vi "begin5RobotsPassGamePlay.vi"(8 "error in (no error)":errorcluster, 10 "Game in":refnum<class "Game.lvclass">, 11 "5RobotsPassGamePlay in":refnum<class "5RobotsPassGamePlay.lvclass">) -> (0 "error out":errorcluster, 1 "Game out":refnum<class "Game.lvclass">, 2 "begin":bool, 3 "5RobotsPassGamePlay out":refnum<class "5RobotsPassGamePlay.lvclass">)   [LabVIEW 2020, in "5RobotsPassGamePlay.lvclass"]
uses:
  5RobotsPassGamePlay.lvclass
  Game_class/Game.lvclass
  Utilities_class/Utilities.lvclass
  Robot_class/roles.ctl
  Referee_class/command_interpreted.ctl
  Team_class/OffensivePlay.ctl
  Game_class/Game.lvclass/Game.ctl
  Playbook_class/Playbook.lvclass/Playbook.ctl
  Team_class/Team.lvclass/Team.ctl
  Referee_class/Referee.lvclass/Referee.ctl
  Object_class/Object.lvclass/Object.ctl
  Events_class/Events.lvclass/Events.ctl
  Robot_class/Robot.lvclass/Robot.ctl
  5RobotsPassGamePlay.lvclass/5RobotsPassGamePlay.ctl
  Write factorPassAlreadyCalculated_.vi
  Playbook_class/Write offensive_plays.vi
  Referee_class/Read command_interpreted.vi
  Team_class/Read OffensivePlay.vi
  Read factorPassAlreadyCalculated_.vi
  Game_class/Read OffensiveTeam.vi
  Game_class/Read Referee.vi
  Game_class/Read BallRef.vi
  Game_class/Read EventsRef.vi
  Events_class/Read enemy_ball_possesion.vi
  Object_class/Read x.vi
  Object_class/Read y.vi
  Team_class/Read RobotRef.vi
  Robot_class/Read dest_x_kick.vi
  Robot_class/Read dest_y_kick.vi
  Playbook_class/Read offensive_plays.vi
  Ball_class/Ball.lvclass
  C:/RoboIME/SSL_AI/Object_class/Object.lvclass
  Ally_class/Ally.lvclass
  C:/RoboIME/SSL_AI/Team_class/Team.lvclass
  Robot_class/Robot.lvclass
  Playbook_class/Playbook.lvclass
  Referee_class/Referee.lvclass
  Events_class/Events.lvclass
  Play_class/Play.lvclass
  TestPlay_class/TestPlay.lvclass
  EnemyPossessionAtEnemyFieldPlay_class/EnemyPossessionAtEnemyFieldPlay.lvclass
  EnemyPossessionAtOurFieldPlay_class/EnemyPossessionAtOurFieldPlay.lvclass
  NormalGamePlay_class/NormalGamePlay.lvclass
  IndirectEnemyPlay_class/IndirectEnemyPlay.lvclass
  PrepareKickoffAllyPlay_class/PrepareKickoffAllyPlay.lvclass
  PrepareKickoffEnemyPlay_class/PrepareKickoffEnemyPlay.lvclass
  KickPenaltyAllyPlay_class/KickPenaltyAllyPlay.lvclass
  PreparePenaltyAllyPlay_class/PreparePenaltyAllyPlay.lvclass
  DirectEnemyPlay_class/DirectEnemyPlay.lvclass
  PreparePenaltyEnemyPlay_class/PreparePenaltyEnemyPlay.lvclass
  BallOutOfFieldPlay_class/BallOutOfFieldPlay.lvclass
  StopOffensivePlay_class/StopOffensivePlay.lvclass
  PassPlay_class/PassPlay.lvclass
  DirectKickPlay_class/DirectKickPlay.lvclass
  HaltPlay_class/HaltPlay.lvclass
  PreparePassPlay_class/PreparePassPlay.lvclass
  PassToStriker_class/PassToStriker.lvclass
  PassTo2ndStriker_class/PassTo2ndStriker.lvclass
  SimplePass_class/SimplePass.lvclass
  PrepareRollToPassPlay_class/PrepareRollToPassPlay.lvclass
  PrepareDoublePassPlay_class/PrepareDoublePassPlay.lvclass
  TableWith2ndStrikerPlay_class/TableWith2ndStrikerPlay.lvclass
  TableWithStrikerPlay_class/TableWithStrikerPlay.lvclass
  PrepareTriplePassPlay_class/PrepareTriplePassPlay.lvclass
  ABCPassPlay_class/ABCPassPlay.lvclass
  PreparePassInGame1_class/PreparePassInGame1.lvclass
  ACBPassPlay_class/ACBPassPlay.lvclass
  PrepareKeeperPassPlay_class/PrepareKeeperPassPlay.lvclass
  KeeperPassToStrikerPlay_class/KeeperPassToStrikerPlay.lvclass
  5RobotsNormalGamePlay_class/5RobotsNormalGamePlay.lvclass
  5RobotsKeeperGame_class/5RobotsKeeperGame.lvclass
  5PreparePassGamePlay_class/5PreparePassGamePlay.lvclass
panel:
  out "DebugGoal":dbl[][](array[numeric])
  out "DebugRobots":dbl[][](array[numeric])
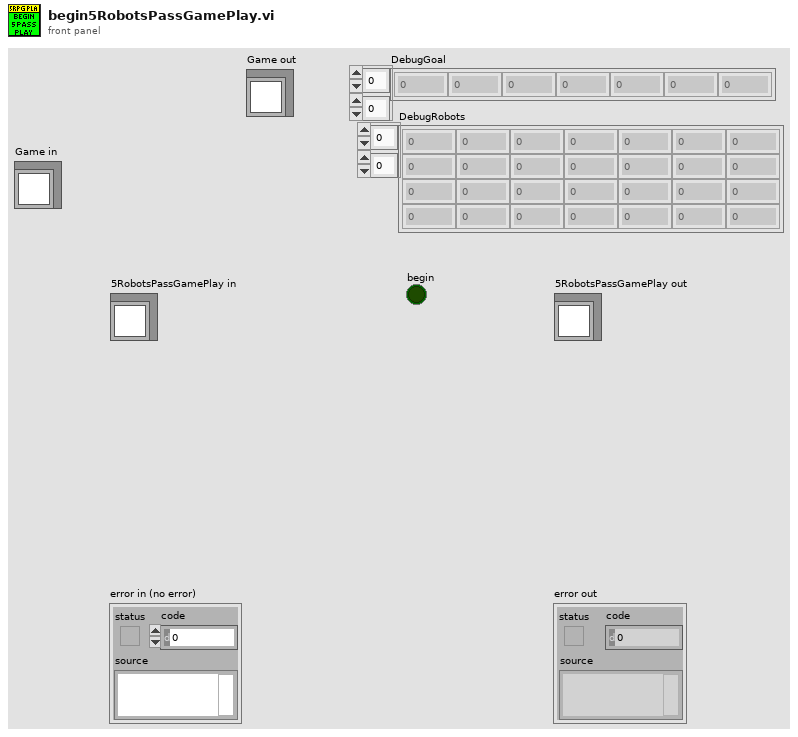
[diagram p1: front panel]
types:
  T1 = typedef "OffensivePlay.ctl" = enum16{"5RobotsPassGamePlay", "5PreparePassGame", "5RobotsKeeperGame", "KeeperPassToStriker", "5RobotsNormalGamePlay", "PrepareKeeperPass", "ACBPass", "ABCPass", "PrepareTriplePass", "TableWithStriker", "TableWith2ndStrikerPlay", "PrepareDoublePass", "PrepareRollToPass", "SimplePass", "PreparePass", "PassToStriker", "BallOutOfField", "PassTo2ndStriker", "StopOffensive", "Prepare Penalty Enemy", "EnemyPossessionAtEnemyField", "EnemyPossesionAtOurField", "TestPlay", "PreparePenaltyAlly", "KickPenaltyAlly", "PrepareKickoffAlly", "PrepareKickoffEnemy", "IndirectEnemy", "DirectEnemy", "PreparePassInGame1", "NormalGame", "DirectKick", "Pass", "Halt", "Timeout", "PassPlay", "PenaltyEnemy"}
  T2 = typedef "command_interpreted.ctl" = enum16{"Goal Ally", "Goal Enemy", "Ball Placement Enemy", "Ball Placement Ally", "Normal Half Time", "Extra Time  Break", "Extra Half Time", "None", "Post Game", "PKA Normal Start", "Prepare Kickoff Ally", "PKE Normal Start", "Prepare Kickoff Enemy", "Force Start", "Halt", "Timeout", "Prepare Penalty Ally", "Prepare Penalty Enemy", "PPA NormalStart", "PPE Normal Start", "Indirect Free Ally", "Direct Free Enemy", "Direct Free Ally", "Indirect Free Enemy", "Stop"}
  T3 = typedef "roles.ctl" = enum16{"SecondMarker", "5Robots5th", "PassBestReceiver", "5Robots4th", "5Robots3rd", "5Robots2nd", "5Robots1st", "PassBestRobot", "WaitPass", "ABCThirdKicker", "ABCFirstKicker", "ABCSecondKicker", "Tabler", "TableFinalizer", "PrepareRollToPassRoller", "PrepareRollToPassReceiver", "SimplePassRoll", "SimplePassRollReceiver", "PenaltyDefense", "PreparePassReceiver 2", "PreparePassReceiver 1", "PassObserver", "Timeout", "Goto", "ZigZag", "None", "BallOutOfField", "DefenderArea", "Duelist", "AttackerStop", "FollowAttacker", "KeeperRole", "KickPenalty", "AttackerAimGoal", "AttackerBlock", "Marker", "Halt", "Shoot", "PassKicker", "PassReceiver", "TestRole", "PenaltyAttacker"}
  T4 = typedef "offensive_plays.ctl" = cluster{"Play":refnum<class "Play.lvclass">, "TestPlay":refnum<class "TestPlay.lvclass">, "EnemyPossessionAtEnemyFieldPlay":refnum<class "EnemyPossessionAtEnemyFieldPlay.lvclass">, "EnemyPossessionAtOurFieldPlay":refnum<class "EnemyPossessionAtOurFieldPlay.lvclass">, "NormalGamePlay":refnum<class "NormalGamePlay.lvclass">, "IndirectEnemyPlay":refnum<class "IndirectEnemyPlay.lvclass">, "PrepareKickoffAllyPlay":refnum<class "PrepareKickoffAllyPlay.lvclass">, "PrepareKickoffEnemyPlay":refnum<class "PrepareKickoffEnemyPlay.lvclass">, "KickPenaltyAllyPlay":refnum<class "KickPenaltyAllyPlay.lvclass">, "PreparePenaltyAllyPlay":refnum<class "PreparePenaltyAllyPlay.lvclass">, "DirectEnemyPlay":refnum<class "DirectEnemyPlay.lvclass">, "PreparePenaltyEnemyPlay":refnum<class "PreparePenaltyEnemyPlay.lvclass">, "BallOutOfFieldPlay":refnum<class "BallOutOfFieldPlay.lvclass">, "StopOffensivePlay":refnum<class "StopOffensivePlay.lvclass">, "PassPlay":refnum<class "PassPlay.lvclass">, "DirectKickPlay":refnum<class "DirectKickPlay.lvclass">, "HaltPlay":refnum<class "HaltPlay.lvclass">, "PreparePassPlay":refnum<class "PreparePassPlay.lvclass">, "PassToStrikerPlay":refnum<class "PassToStriker.lvclass">, "PassTo2ndStrikerPlay":refnum<class "PassTo2ndStriker.lvclass">, "SimplePassPlay":refnum<class "SimplePass.lvclass">, "PrepareRollToPassPlay":refnum<class "PrepareRollToPassPlay.lvclass">, "PrepareDoublePassPlay":refnum<class "PrepareDoublePassPlay.lvclass">, "TableWith2ndStrikerPlay":refnum<class "TableWith2ndStrikerPlay.lvclass">, "TableWithStrikerPlay":refnum<class "TableWithStrikerPlay.lvclass">, "PrepareTriplePassPlay":refnum<class "PrepareTriplePassPlay.lvclass">, "ABCPassPlay":refnum<class "ABCPassPlay.lvclass">, "PreparePassInGame1":refnum<class "PreparePassInGame1.lvclass">, "ACBPassPlay":refnum<class "ACBPassPlay.lvclass">, "PrepareKeeperPassPlay":refnum<class "PrepareKeeperPassPlay.lvclass">, "KeeperPassToStrikerPlay":refnum<class "KeeperPassToStrikerPlay.lvclass">, "SimplePass":refnum<class "SimplePass.lvclass">, "SimplePass 2":refnum<class "SimplePass.lvclass">, "5RobotsNormalGamePlay":refnum<class "5RobotsNormalGamePlay.lvclass">, "5RobotsPassGamePlay":refnum<class "5RobotsPassGamePlay.lvclass">, "5RobotsKeeperGame":refnum<class "5RobotsKeeperGame.lvclass">, "5PreparePassGamePlay":refnum<class "5PreparePassGamePlay.lvclass">}
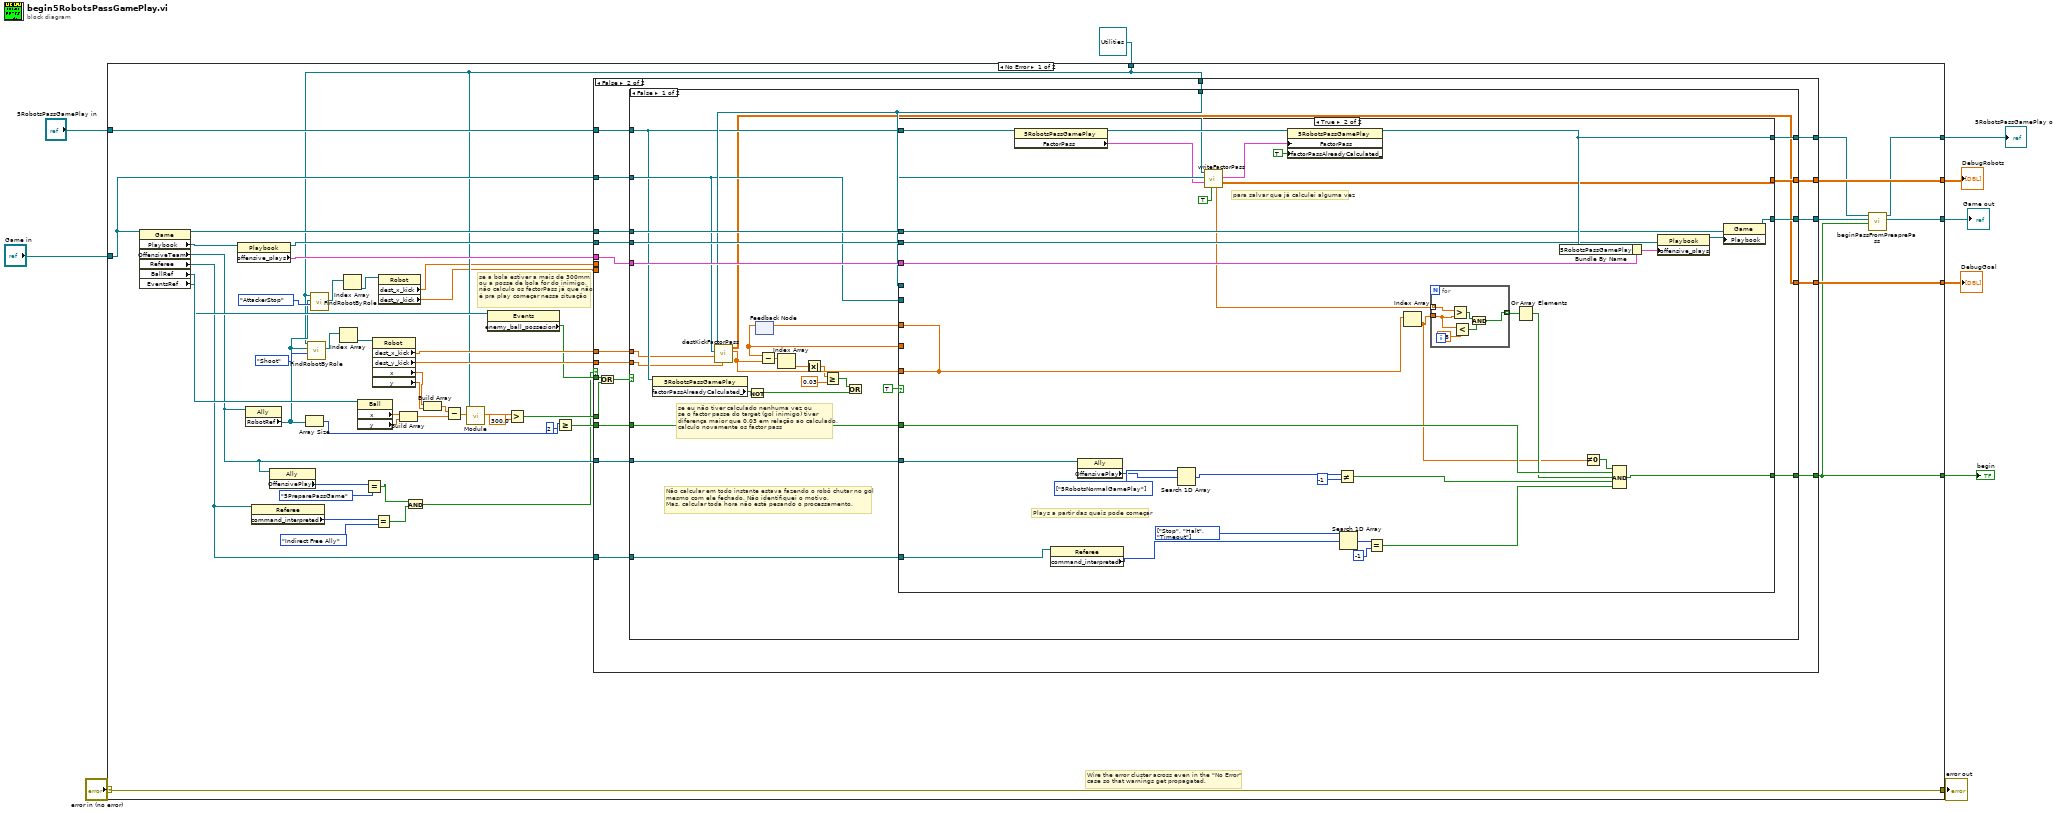
[diagram p0: block diagram]
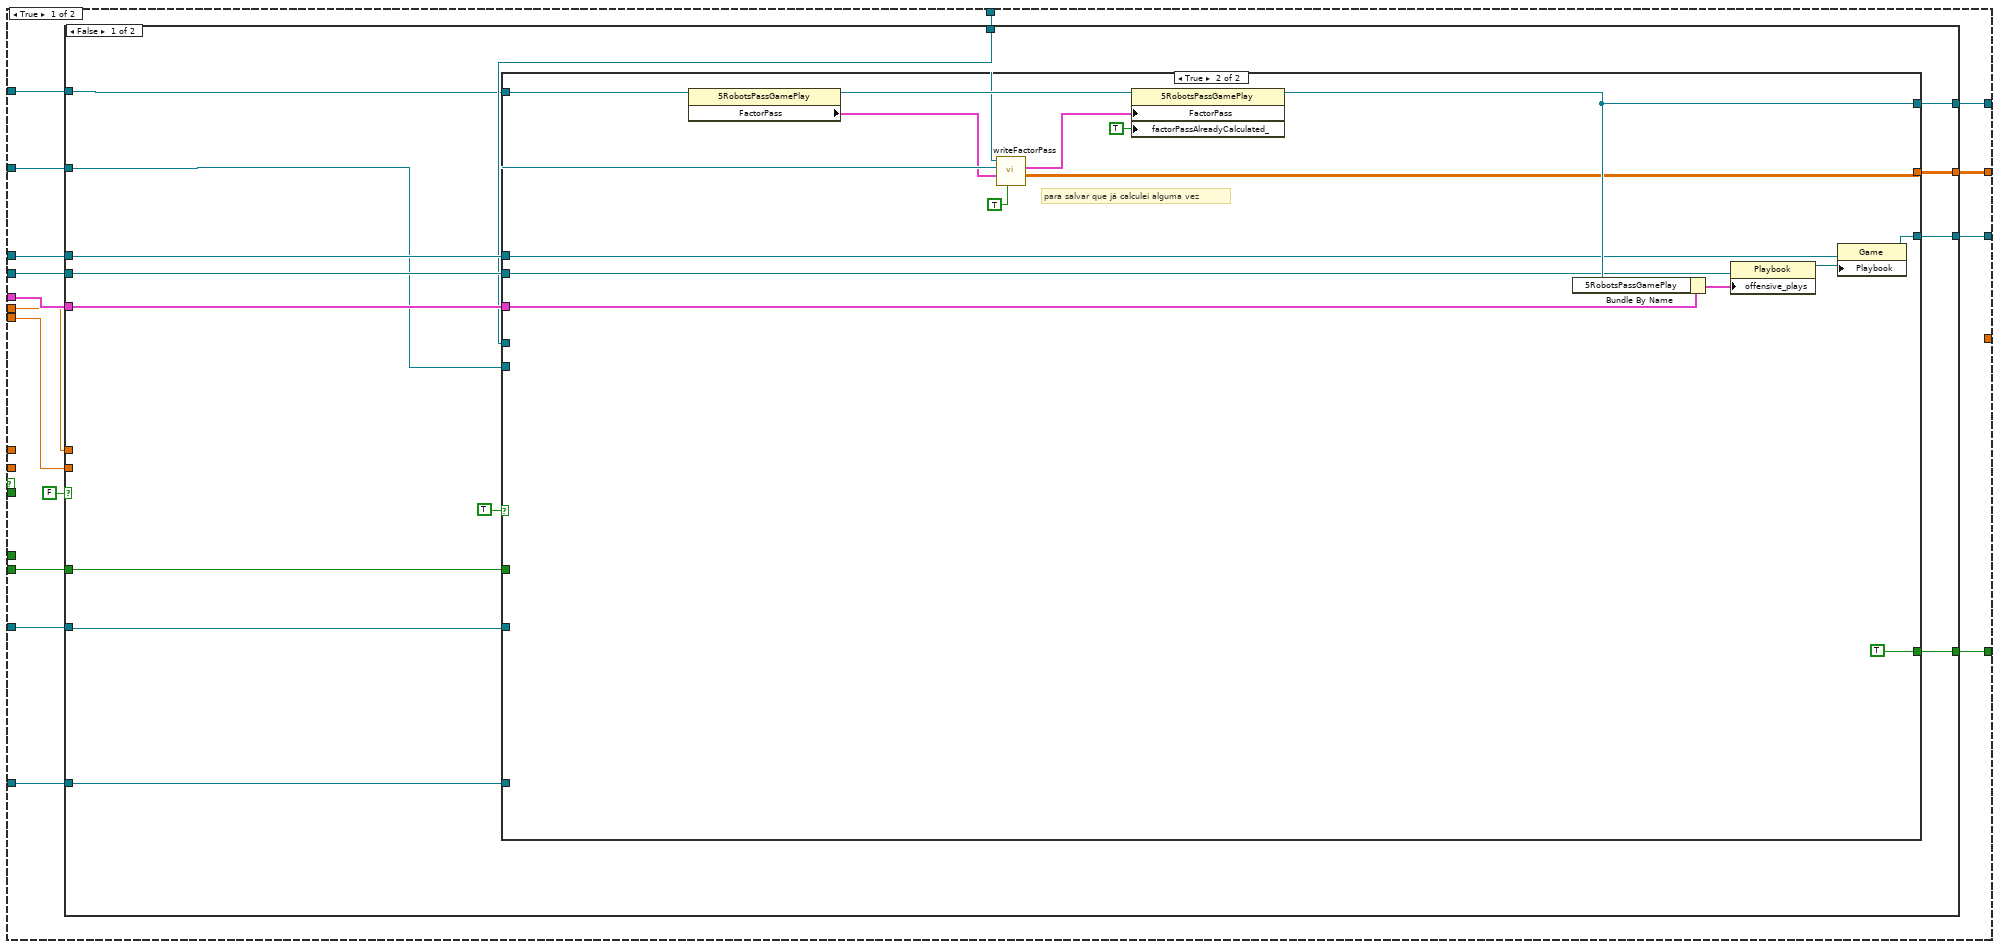
[diagram p2: hidden frame]
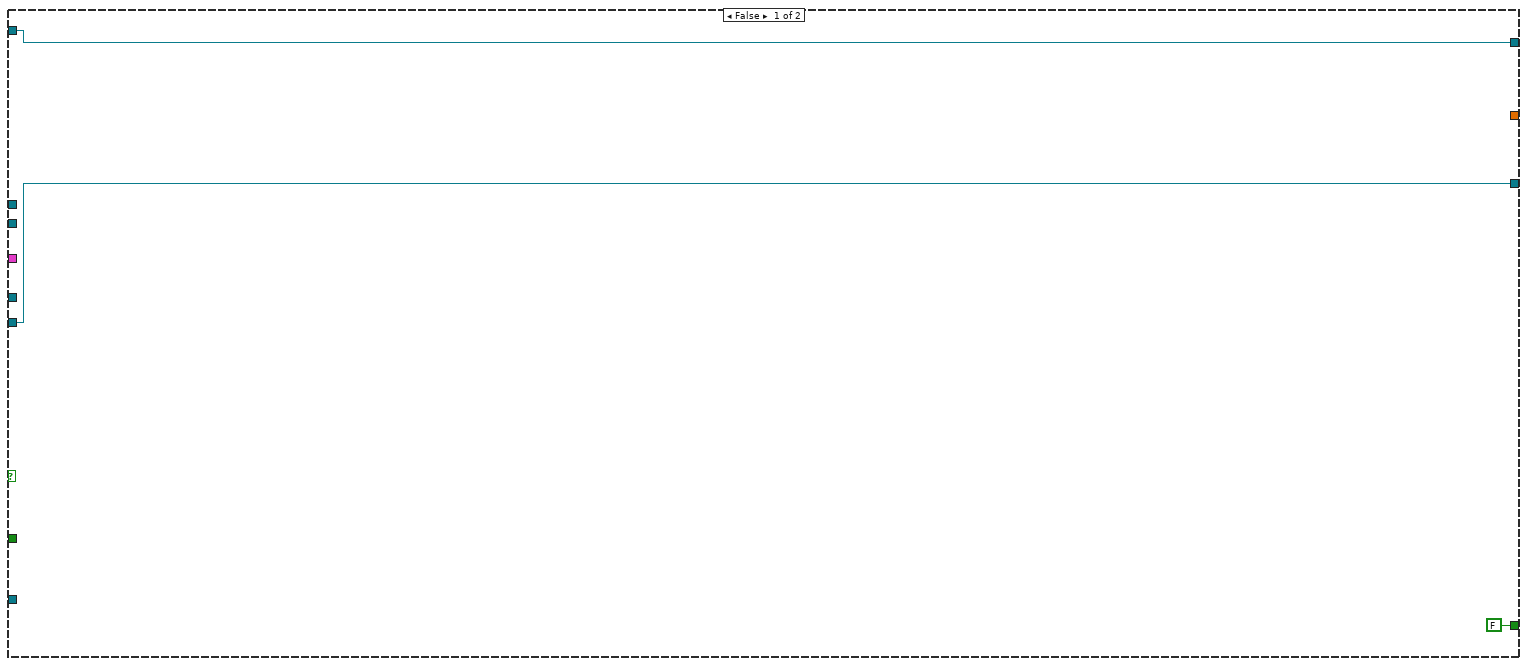
[diagram p3: hidden frame]
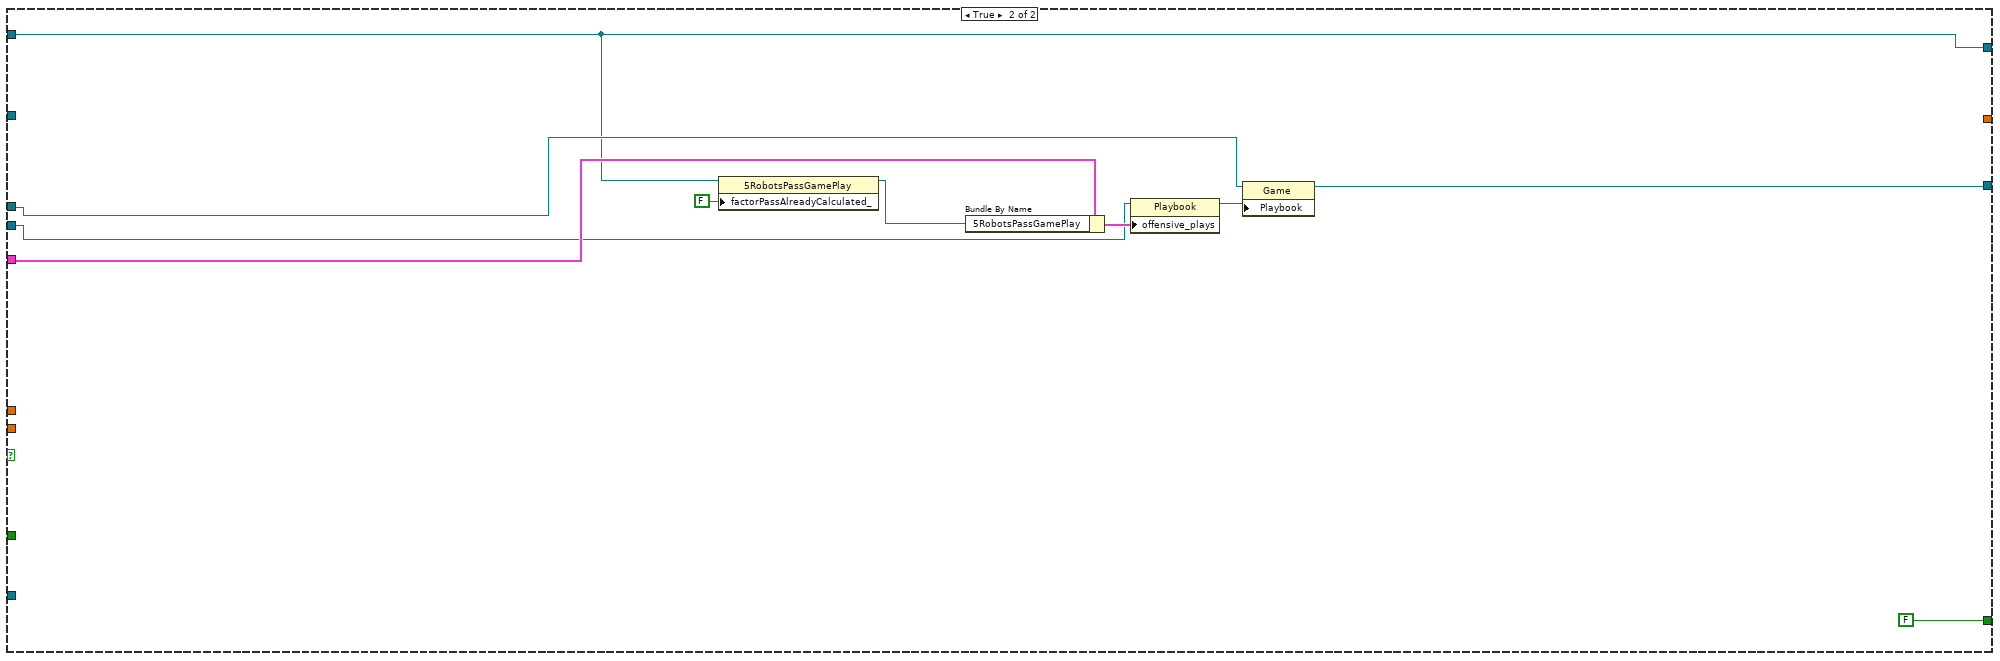
[diagram p4: hidden frame]
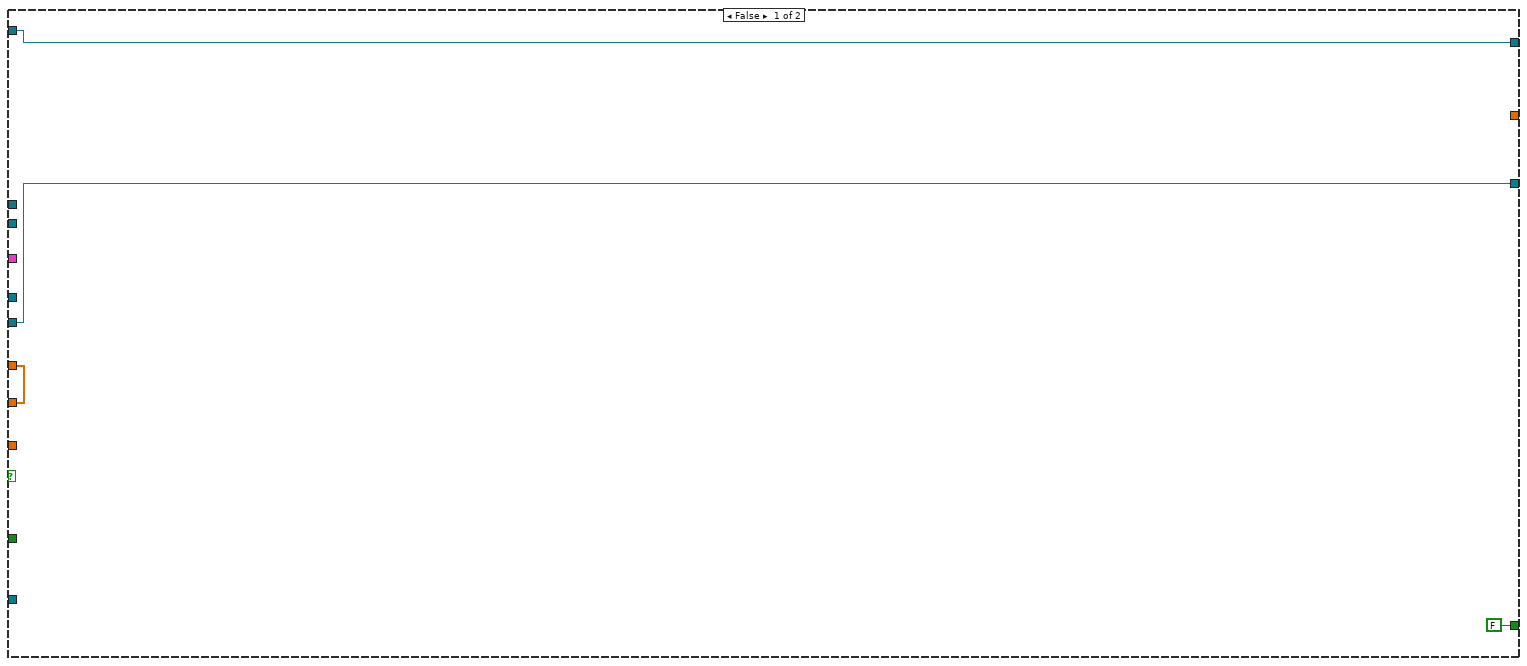
[diagram p5: hidden frame]
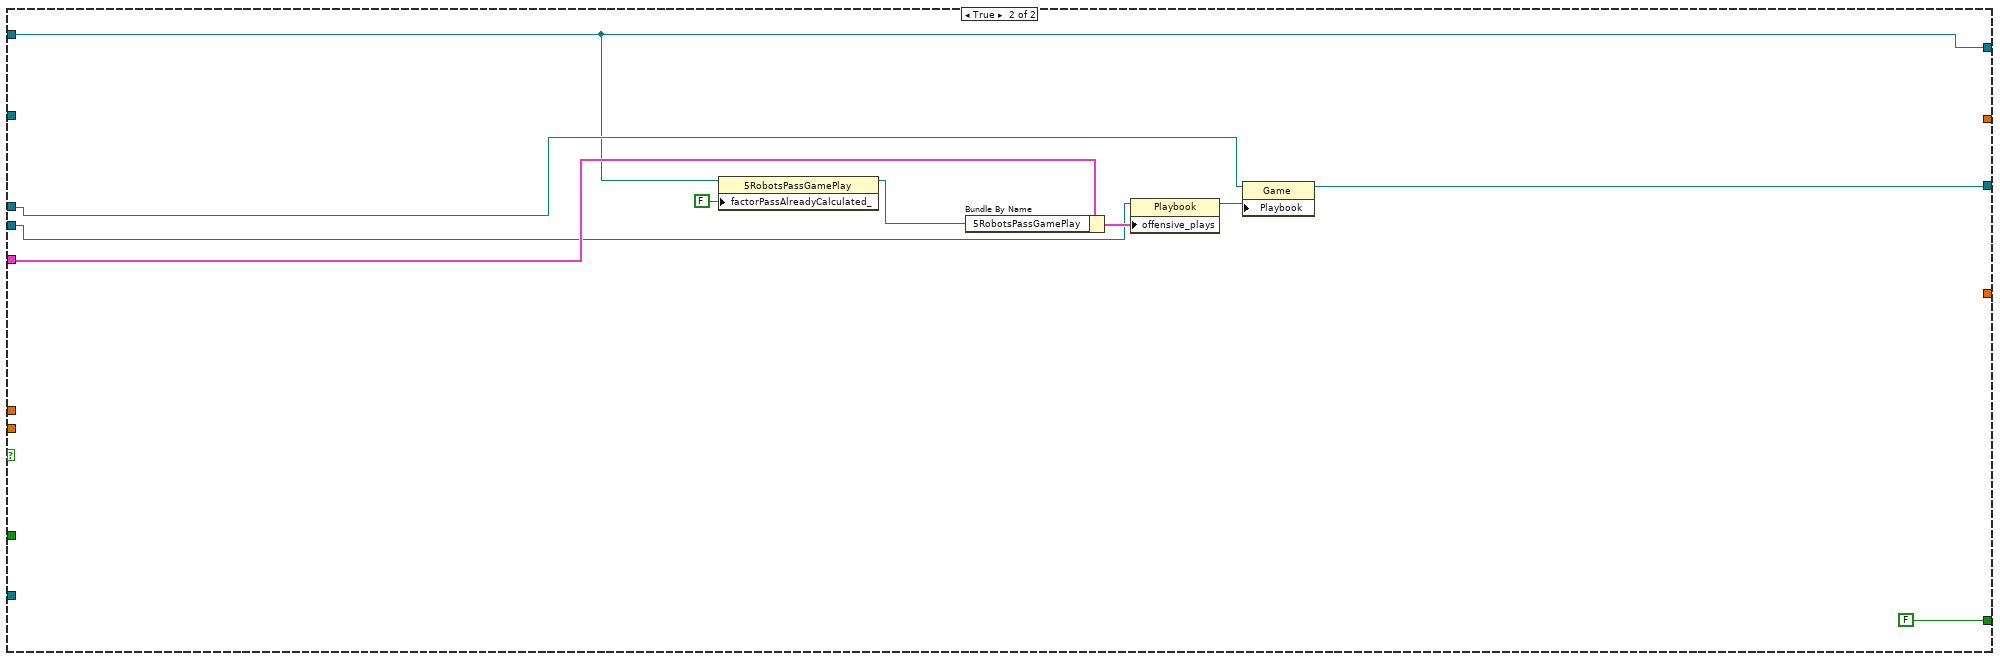
[diagram p6: hidden frame]
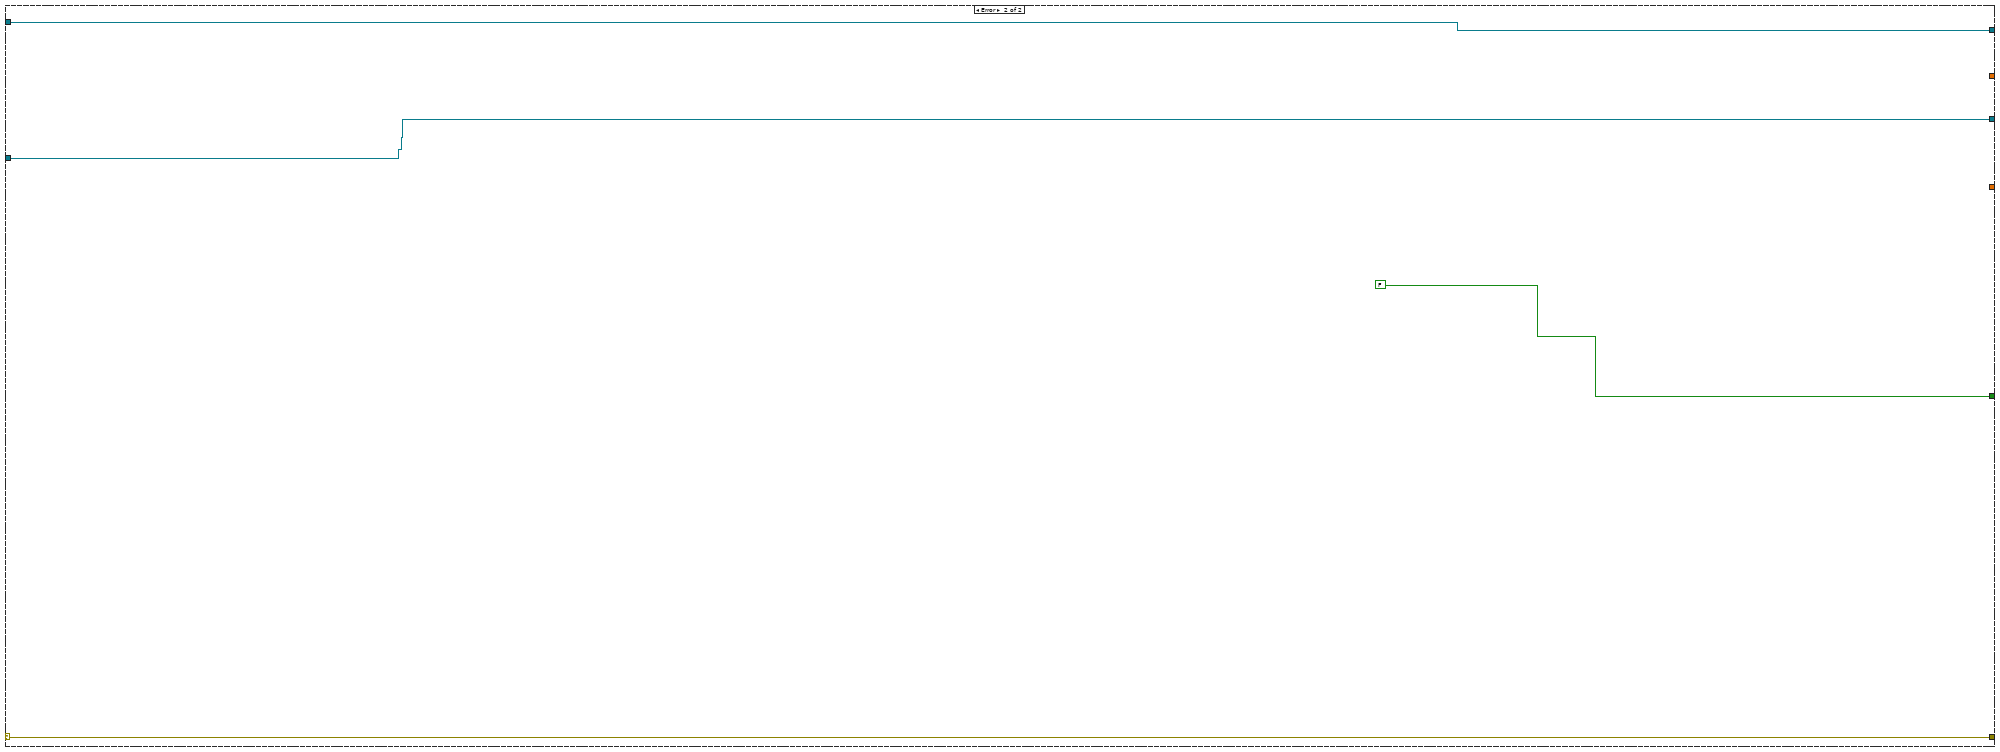
[diagram p7: hidden frame]
diagram:
  n1 = case shown="No Error" "error in (no error)" {
    selector: "error in (no error)" -> [w61 w227]
    tunnel: [w61 w227] -> w9
    tunnel: [w11 w226] -> w7
    tunnel: "5RobotsPassGamePlay in" -> [w60 w226]
    tunnel: [w13 FALSE] -> w6
    tunnel: [w15 w224] -> w4
    tunnel: "Game in" -> [w35 w224]
    tunnel: refnum<class "Utilities.lvclass"> refnum ("Utilities in") -> [w29 _]
    tunnel: [w52 _] -> w2
    tunnel: [w36 _] -> w1
    frame No Error {
      # "se a bola estiver a mais de 300mm\nou a posse de bola for do inimigo,\nnão calculo os factorPass já que não\né pra play começar nessa situação"
      # "Wire the error cluster across even in the \"No Error\"\ncase so that warnings get propagated."
      n2 = property class="Game"(reference=w35) -> (reference out=w53:refnum<class "Game.lvclass">, "Playbook"=w56:refnum<class "Playbook.lvclass">, "OffensiveTeam"=w21:refnum<class "Ally.lvclass">, "Referee"=w24:refnum<class "Referee.lvclass">, "BallRef"=w44:refnum<class "Ball.lvclass">, "EventsRef"=w33:refnum<class "Events.lvclass">)  [unwired: 1 in, 1 out]
      n3 = property class="Playbook"(reference=w56) -> (reference out=w54:refnum<class "Playbook.lvclass">, "offensive_plays"=w55:T4)  [unwired: 1 in, 1 out]
      n4 = property class="Ally"(reference=w21) -> ("RobotRef"=w30:refnum<class "Robot.lvclass">[])  [unwired: 1 in, 2 out]
      n5 = property class="Referee"(reference=w24) -> ("command_interpreted"=w23:T2)  [unwired: 1 in, 2 out]
      n6 = property class="Ally"(reference=w21) -> ("OffensivePlay"=w20:T1)  [unwired: 1 in, 2 out]
      n7 = Array Size(array=w30) -> (size(s)=w59:i32)
      n8 = call "FindRobotByRole.vi"("role"=roles."Shoot", "RobotRef"=w30, "Utilities in"=w29) -> ("Robots"=w50:refnum<class "Robot.lvclass">[])  [unwired: 6 in, 2 out]
      n9 = call "FindRobotByRole.vi"("role"=roles."AttackerStop", "RobotRef"=w30, "Utilities in"=w29) -> ("Robots"=w28:refnum<class "Robot.lvclass">[])  [unwired: 6 in, 2 out]
      n10 = Index Array(array=w50) -> (element=w49:refnum<class "Robot.lvclass">)  [unwired: 1 in]
      n11 = Index Array(array=w28) -> (element=w27:refnum<class "Robot.lvclass">)  [unwired: 1 in]
      n12 = property class="Ball"(reference=w44) -> ("x"=w43:dbl, "y"=w42:dbl)  [unwired: 1 in, 2 out]
      n13 = Equal?(x=w20, y=OffensivePlay."5PreparePassGame") -> (x = y?=w17:bool)
      n14 = property class="Robot"(reference=w49) -> ("dest_x_kick"=w48:dbl, "dest_y_kick"=w47:dbl, "x"=w46:dbl, "y"=w45:dbl)  [unwired: 1 in, 2 out]
      n15 = Equal?(x=w23, y=command_interpreted."Indirect Free Ally") -> (x = y?=w18:bool)
      n16 = property class="Robot"(reference=w27) -> ("dest_x_kick"=w26:dbl, "dest_y_kick"=w25:dbl)  [unwired: 1 in, 2 out]
      n17 = Build Array(w43, w42) -> (w41:dbl[])
      n18 = And(x=w17, y=w18) -> (x .and. y?=w16:bool)
      n19 = Build Array(w46, w45) -> (w40:dbl[])
      n20 = Subtract(x=w40, y=w41) -> (x-y=w39:dbl[])
      n21 = call "Module.vi"("2D vector"=w39, "Utilities in"=w29) -> ("Modulo"=w38:dbl)  [unwired: 7 in, 2 out]
      n22 = property class="Events"(reference=w33) -> ("enemy_ball_possesion"=w32:bool)  [unwired: 1 in, 2 out]
      n23 = Greater?(x=w38, y=300.0) -> (0:w34:bool)
      n24 = Greater Or Equal?(x=w59, y=2) -> (x >= y?=w57:bool)
      n25 = case shown="False" w16 {
        tunnel: w60 -> [w77 w140]
        tunnel: w21 -> [w76 w139]
        tunnel: w57 -> [w75 w138]
        tunnel: w24 -> [w74 w137]
        tunnel: [w73 w136] -> w13
        tunnel: w55 -> [w72 w135]
        tunnel: [w71 w134] -> w12
        tunnel: w54 -> [w70 w133]
        tunnel: w53 -> [w69 w132]
        tunnel: [w68 w131] -> w14
        tunnel: [_ w130] -> w52
        tunnel: w48 -> [_ w129]
        tunnel: w47 -> [_ w128]
        tunnel: [w67 w127] -> w36
        tunnel: w29 -> [w66 w126]
        tunnel: w35 -> [w65 w125]
        tunnel: w34 -> [_ w124]
        tunnel: w32 -> [_ w122]
        tunnel: w26 -> [w64 _]
        tunnel: w25 -> [w63 _]
        frame True {
          n26 = case shown="False" FALSE {
            tunnel: w77 -> [w79 w114]
            tunnel: w76 -> [w91 _]
            tunnel: w75 -> [w90 _]
            tunnel: w74 -> [w89 _]
            tunnel: [w88 FALSE] -> w73
            tunnel: w72 -> [w87 w117]
            tunnel: [w86 w114] -> w71
            tunnel: w70 -> [w85 w116]
            tunnel: w69 -> [w84 w115]
            tunnel: [w83 w112] -> w68
            tunnel: w64 -> [_ _]
            tunnel: w63 -> [_ _]
            tunnel: [w82 _] -> w67
            tunnel: w66 -> [w81 _]
            tunnel: w65 -> [w80 _]
            frame False {
              n27 = case shown="True" TRUE {
                tunnel: w79 -> [w92 w111]
                tunnel: w91 -> [_ _]
                tunnel: w90 -> [_ _]
                tunnel: w89 -> [_ _]
                tunnel: [FALSE TRUE] -> w88
                tunnel: w87 -> [_ w109]
                tunnel: [w92 w108] -> w86
                tunnel: w85 -> [_ w107]
                tunnel: w84 -> [_ w105]
                tunnel: [w93 w103] -> w83
                tunnel: [_ w101] -> w82
                tunnel: w81 -> [_ w100]
                tunnel: w80 -> [w93 w98]
                frame False {
                }
                frame True {
                  # "para salvar que já calculei alguma vez"
                  n28 = property class="5RobotsPassGamePlay"(reference=w111) -> (reference out=w110:refnum<class "5RobotsPassGamePlay.lvclass">, "FactorPass"=w97:cluster{"id":dbl[], "value":dbl[]})  [unwired: 1 in, 1 out]
                  n29 = call "writeFactorPass.vi"("Pass?"=TRUE, "FactorPass in"=w97, "Game in"=w98, "Utilities in"=w100) -> ("Debug"=w101:dbl[][], "FactorPass out"=w102:cluster{"id":dbl[], "value":dbl[]})  [unwired: 3 in, 3 out]
                  n30 = property class="5RobotsPassGamePlay"(reference=w110, "FactorPass"=w102, "factorPassAlreadyCalculated_"=TRUE) -> (reference out=w108:refnum<class "5RobotsPassGamePlay.lvclass">)  [unwired: 1 in, 1 out]
                  n31 = Bundle By Name(cluster=w109, "5RobotsPassGamePlay"=w108) -> (w106:T4)
                  n32 = property class="Playbook"(reference=w107, "offensive_plays"=w106) -> (reference out=w104:refnum<class "Playbook.lvclass">)  [unwired: 1 in, 1 out]
                  n33 = property class="Game"(reference=w105, "Playbook"=w104) -> (reference out=w103:refnum<class "Game.lvclass">)  [unwired: 1 in, 1 out]
                }
              }
            }
            frame True {
              n34 = property class="5RobotsPassGamePlay"(reference=w114, "factorPassAlreadyCalculated_"=FALSE) -> (reference out=w113:refnum<class "5RobotsPassGamePlay.lvclass">)  [unwired: 1 in, 1 out]
              n35 = Bundle By Name(cluster=w117, "5RobotsPassGamePlay"=w113) -> (w120:T4)
              n36 = property class="Playbook"(reference=w116, "offensive_plays"=w120) -> (reference out=w119:refnum<class "Playbook.lvclass">)  [unwired: 1 in, 1 out]
              n37 = property class="Game"(reference=w115, "Playbook"=w119) -> (reference out=w112:refnum<class "Game.lvclass">)  [unwired: 1 in, 1 out]
            }
          }
        }
        frame False {
          n38 = Or(x=w122, y=w124) -> (x .or. y?=w123:bool)
          n39 = case shown="False" w123 {
            tunnel: w140 -> [w155 w216]
            tunnel: w139 -> [w167 _]
            tunnel: w138 -> [w166 _]
            tunnel: w137 -> [w165 _]
            tunnel: [w164 FALSE] -> w136
            tunnel: w135 -> [w163 w219]
            tunnel: [w162 w216] -> w134
            tunnel: w133 -> [w161 w218]
            tunnel: w132 -> [w160 w217]
            tunnel: [w159 w214] -> w131
            tunnel: [w152 _] -> w130
            tunnel: w129 -> [w153 _]
            tunnel: w128 -> [w154 _]
            tunnel: [w158 _] -> w127
            tunnel: w126 -> [w157 _]
            tunnel: w125 -> [w156 _]
            frame False {
              # "Não calcular em todo instante estava fazendo o robô chutar no gol\nmesmo com ele fechado. Não identifiquei o motivo.\nMas, calcular toda hora não está pesando o processamento."
              # "se eu não tiver calculado nenhuma vez ou\nse o factor passe do target (gol inimigo) tiver\ndiferença maior que 0,03 em relação ao calculado,\ncalculo novamente os factor pass"
              n40 = property class="5RobotsPassGamePlay"(reference=w155) -> ("factorPassAlreadyCalculated_"=w143:bool)  [unwired: 1 in, 2 out]
              n41 = call "destKickFactorPass.vi"("dest_y_kick"=w154, "dest_x_kick"=w153, "Game in"=w156, "Utilities in"=w157) -> ("FactorPass"=w149:dbl[], "Debug"=w152:dbl[][])  [unwired: 6 in]
              n42 = Not(x=w143) -> (.not. x?=w142:bool)
              n43 = feedback #1() -> (w150:dbl[])  [unwired: 1 in]
              n44 = Subtract(x=w150, y=w149) -> (x-y=w148:dbl[])
              n45 = Index Array(array=w148) -> (element=w147:dbl)  [unwired: 1 in]
              n46 = Absolute Value(x=w147) -> (abs(x)=w146:dbl)
              n47 = Greater Or Equal?(x=w146, y=0.03) -> (x >= y?=w144:bool)
              n48 = Or(x=w144, y=w142) -> ()  [unwired: 1 out]
              n49 = case shown="True" TRUE {
                tunnel: w155 -> [w168 w207]
                tunnel: w167 -> [_ w205]
                tunnel: w166 -> [_ w204]
                tunnel: w165 -> [_ w194]
                tunnel: [FALSE w192] -> w164
                tunnel: w163 -> [_ w190]
                tunnel: [w168 w189] -> w162
                tunnel: w161 -> [_ w188]
                tunnel: w160 -> [_ w186]
                tunnel: [w169 w184] -> w159
                tunnel: [_ w179] -> w158
                tunnel: w157 -> [_ w177]
                tunnel: w156 -> [w169 w175]
                tunnel: w149 -> [_ w174]
                tunnel: [w170 w174] -> w151
                tunnel: w150 -> [w170 _]
                frame False {
                }
                frame True {
                  w197 = T2[] [enum."Stop", enum."Halt", enum."Timeout"] items=["Goal Ally", "Goal Enemy", "Ball Placement Enemy", "Ball Placement Ally", "Normal Half Time", "Extra Time  Break", "Extra Half Time", "None", "Post Game", "PKA Normal Start", "Prepare Kickoff Ally", "PKE Normal Start", "Prepare Kickoff Enemy", "Force Start", "Halt", "Timeout", "Prepare Penalty Ally", "Prepare Penalty Enemy", "PPA NormalStart", "PPE Normal Start", "Indirect Free Ally", "Direct Free Enemy", "Direct Free Ally", "Indirect Free Enemy", "Stop"] ("1D array")
                  w202 = T1[] [enum."5RobotsNormalGamePlay"] items=["5RobotsPassGamePlay", "5PreparePassGame", "5RobotsKeeperGame", "KeeperPassToStriker", "5RobotsNormalGamePlay", "PrepareKeeperPass", "ACBPass", "ABCPass", "PrepareTriplePass", "TableWithStriker", "TableWith2ndStrikerPlay", "PrepareDoublePass", "PrepareRollToPass", "SimplePass", "PreparePass", "PassToStriker", "BallOutOfField", "PassTo2ndStriker", "StopOffensive", "Prepare Penalty Enemy", "EnemyPossessionAtEnemyField", "EnemyPossesionAtOurField", "TestPlay", "PreparePenaltyAlly", "KickPenaltyAlly", "PrepareKickoffAlly", "PrepareKickoffEnemy", "IndirectEnemy", "DirectEnemy", "PreparePassInGame1", "NormalGame", "DirectKick", "Pass", "Halt", "Timeout", "PassPlay", "PenaltyEnemy"] ("Array")
                  # "para salvar que já calculei alguma vez"
                  # "Plays a partir das quais pode começar"
                  n50 = property class="5RobotsPassGamePlay"(reference=w207) -> (reference out=w191:refnum<class "5RobotsPassGamePlay.lvclass">, "FactorPass"=w173:cluster{"id":dbl[], "value":dbl[]})  [unwired: 1 in, 1 out]
                  n51 = property class="Referee"(reference=w194) -> ("command_interpreted"=w198:T2)  [unwired: 1 in, 2 out]
                  n52 = property class="Ally"(reference=w205) -> ("OffensivePlay"=w183:T1)  [unwired: 1 in, 2 out]
                  n53 = Search 1D Array(1D array=w202, element=w183) -> (index of element=w201:i32)  [unwired: 1 in]
                  n54 = call "writeFactorPass.vi"("Pass?"=TRUE, "FactorPass in"=w173, "Game in"=w175, "Utilities in"=w177) -> ("Debug"=w179:dbl[][], "FactorPass out"=w180:cluster{"id":dbl[], "value":dbl[]}, "FactorPass"=w178:dbl[])  [unwired: 3 in, 2 out]
                  n55 = property class="5RobotsPassGamePlay"(reference=w191, "FactorPass"=w180, "factorPassAlreadyCalculated_"=TRUE) -> (reference out=w189:refnum<class "5RobotsPassGamePlay.lvclass">)  [unwired: 1 in, 1 out]
                  n56 = Not Equal?(x=w201, y=-1) -> (x != y?=w199:bool)
                  n57 = Search 1D Array(1D array=w197, element=w198) -> (index of element=w196:i32)  [unwired: 1 in]
                  n58 = Equal?(x=w196, y=-1) -> (x = y?=w203:bool)
                  n59 = Index Array(array=w174) -> (element=w181:dbl)  [unwired: 1 in]
                  n60 = for {
                    tunnel: w178 -> [w213] mode=indexing
                    tunnel: [w209] -> w206 mode=indexing
                    tunnel: w181 -> [w208]
                    n61 = Greater?(x=w213, y=w208) -> (0:w210:bool)
                    n62 = Less?(x=w208, y=0.8) -> (x < y?=w211:bool)
                    n63 = And(x=w210, y=w211) -> (x .and. y?=w209:bool)
                  }
                  n64 = Or Array Elements(Boolean array=w206) -> (logical OR=w193:bool)
                  n65 = Bundle By Name(cluster=w190, "5RobotsPassGamePlay"=w189) -> (w187:T4)
                  n66 = Not Equal To 0?(x=w181) -> (x != 0?=w182:bool)
                  n67 = Compound Arithmetic op=AND(w182, w204, w193, w199, w203) -> (w192:bool)
                  n68 = property class="Playbook"(reference=w188, "offensive_plays"=w187) -> (reference out=w185:refnum<class "Playbook.lvclass">)  [unwired: 1 in, 1 out]
                  n69 = property class="Game"(reference=w186, "Playbook"=w185) -> (reference out=w184:refnum<class "Game.lvclass">)  [unwired: 1 in, 1 out]
                }
              }
              n70 = feedback-in #1(w151) -> ()
            }
            frame True {
              n71 = property class="5RobotsPassGamePlay"(reference=w216, "factorPassAlreadyCalculated_"=FALSE) -> (reference out=w215:refnum<class "5RobotsPassGamePlay.lvclass">)  [unwired: 1 in, 1 out]
              n72 = Bundle By Name(cluster=w219, "5RobotsPassGamePlay"=w215) -> (w222:T4)
              n73 = property class="Playbook"(reference=w218, "offensive_plays"=w222) -> (reference out=w221:refnum<class "Playbook.lvclass">)  [unwired: 1 in, 1 out]
              n74 = property class="Game"(reference=w217, "Playbook"=w221) -> (reference out=w214:refnum<class "Game.lvclass">)  [unwired: 1 in, 1 out]
            }
          }
        }
      }
      n75 = call "beginPassFromPreaprePass.vi"("begin?"=w13, "Game in"=w14, "5RobotsPassGamePlay in"=w12) -> ("Game out"=w15:refnum<class "Game.lvclass">, "5RobotsPassGamePlay out"=w11:refnum<class "5RobotsPassGamePlay.lvclass">)  [unwired: 6 in, 1 out]
    }
    frame Error {
    }
  }
  "error out" <- w9
  "5RobotsPassGamePlay out" <- w7
  "begin" <- w6
  "Game out" <- w4
  "DebugGoal" <- w2
  "DebugRobots" <- w1
